vi "BuildingGreyLevelDataBase.vi"(8 "error in (no error)":errorcluster, 9 "ConfDB":T1={"NumberOfImages"=0, "NoImages2SaveAroundFreeze"=0, "Path"=path "", "NameOfPartialFile"="", "StartIndex"=0, "NumberOfStdTol"=0, "Detla t (sec)"=0, "Number of images for baseline"=10, "Temperature File Name"="", "Score"=15.0, "Index number of Files"=[]}, 10 "Droplet Bounding Box":cluster{"x":sgl, "y":sgl}[][](array[cluster]), 11 "Image Ref In":T2) -> (0 "error out":errorcluster, 1 "GreyLevel Drops and time":dbl[][](array[numeric]), 2 "Rel Time (s)":u32[](array[numeric]), 3 "Refnum out":T2(plugin-control), 4 "Greylevel deriv per drop per time":dbl[][](array[numeric]))   [LabVIEW 2013]
doc: "Go over all images and retrieve Grey level of each drop and the difference between the i+1 and i image"
uses:
  <vilib>/vision/Image Controls.llb/IMAQ Image.ctl
  DB/ConfDB.ctl
panel:
  out "Numeric":i32
  out "Index":i32
  out "Time(s)":i32
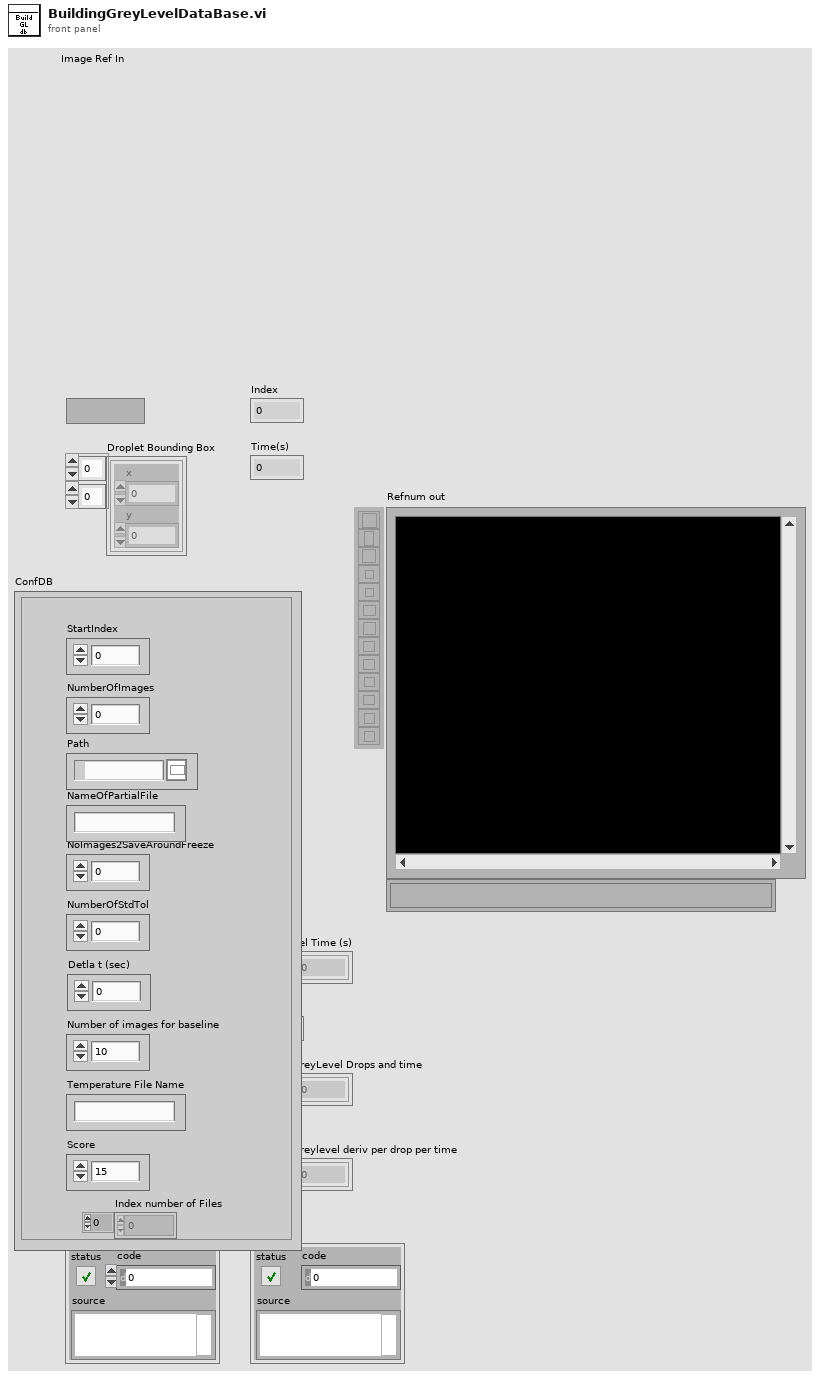
[diagram p1: front panel]
types:
  T1 = typedef "ConfDB.ctl" = cluster{"NumberOfImages":i32, "NoImages2SaveAroundFreeze":i32, "Path":path, "NameOfPartialFile":string, "StartIndex":i32, "NumberOfStdTol":i32, "Detla t (sec)":i32, "Number of images for baseline":i32, "Temperature File Name":string, "Score":dbl, "Index number of Files":i32[]}
  T2 = typedef "IMAQ Image.ctl" = refnum<image>
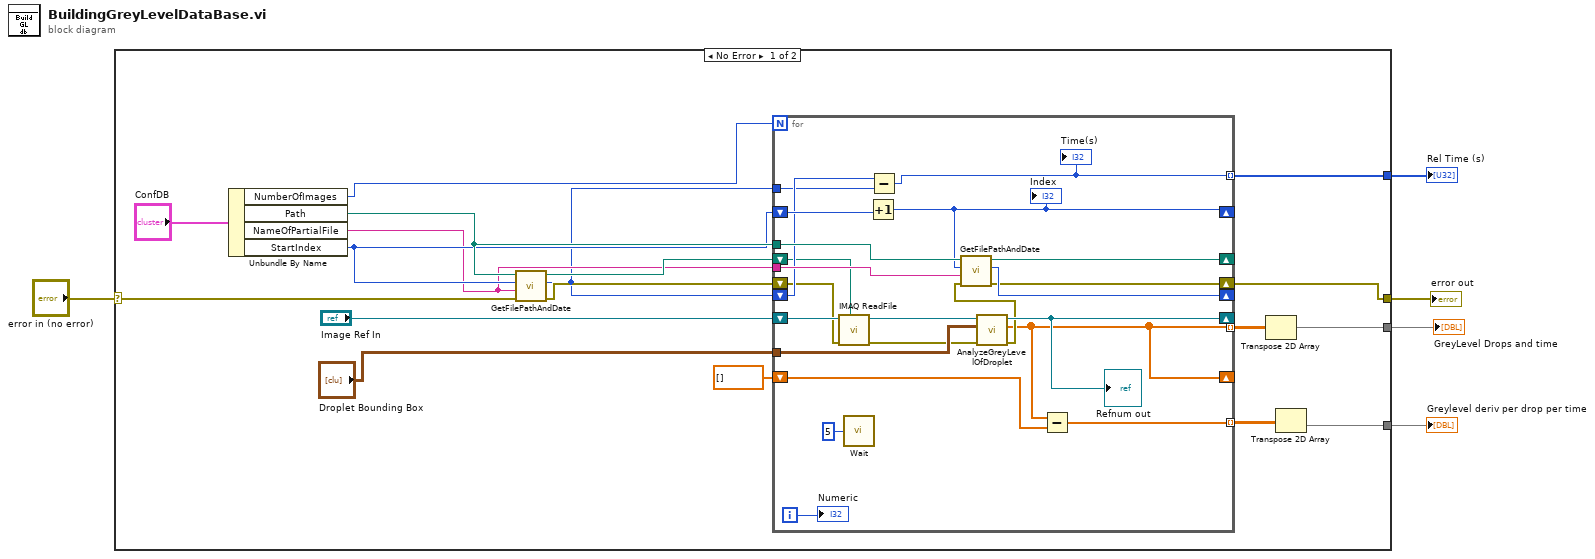
[diagram p0: block diagram]
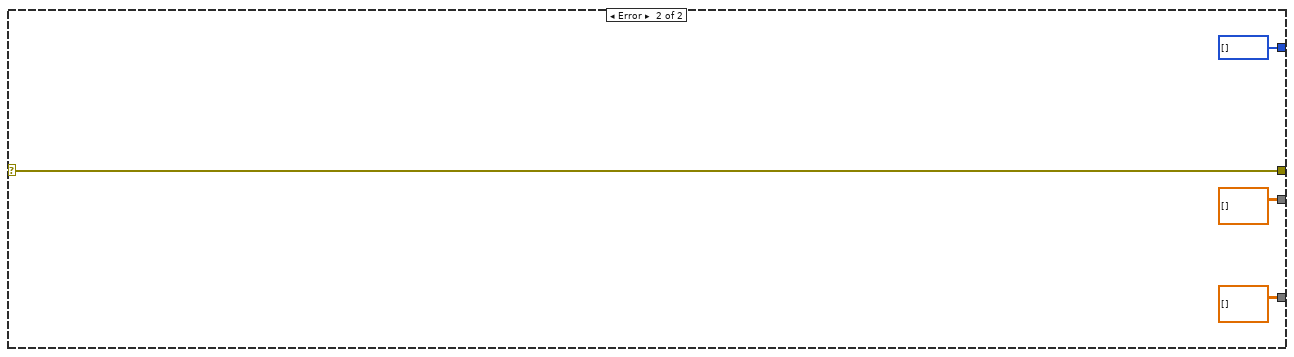
[diagram p2: hidden frame]
diagram:
  n1 = case shown="No Error" "error in (no error)" {
    selector: "error in (no error)" -> [w8 w48]
    tunnel: [w23 dbl[][] []] -> w5
    tunnel: [w21 u32[] []] -> w4
    tunnel: [w19 dbl[][] []] -> w3
    tunnel: [w7 w48] -> w1
    frame No Error {
      n2 = Unbundle By Name("ConfDB") -> ("NumberOfImages"=w18:i32, "Path"=w15:path, "NameOfPartialFile"=w10:string, "StartIndex"=w11:i32)
      n3 = call "GetFilePathAndDate.vi"("error in (no error)"=w8, "String"=w10, "Index"=w11, "Path"=w15) -> ("error out"=w17:errorcluster, "creation date"=w9:u32, "file out"=w14:path)  [unwired: 5 in]
      n4 = for {
        N: w18 -> [_]
        shift-right: [w42] -> _
        shift-left: w11 -> [w46]
        tunnel: [w45] -> w21 mode=indexing
        tunnel: w15 -> [w44]
        tunnel: w10 -> [w43]
        shift-right: [w41] -> _
        shift-left: w14 -> [w35]
        shift-right: [w40] -> _
        shift-left: w9 -> [w39]
        tunnel: w9 -> [w32]
        tunnel: "Droplet Bounding Box" -> [w37]
        shift-right: [w31] -> _
        shift-left: "Image Ref In" -> [w36]
        tunnel: [w26] -> w20 mode=indexing
        shift-right: [w26] -> _
        shift-left: dbl[] [] ("GreyLevelArray") -> [w25]
        shift-right: [w27] -> w7
        shift-left: w17 -> [w30]
        tunnel: [w24] -> w22 mode=indexing
        i -> [w33]
        n5 = call "IMAQ ReadFile"("File Path"=w35, "error in (no error)"=w30, "Image"=w36) -> ("error out"=w29:errorcluster, "Image Out"=w34:T2)  [unwired: 2 in, 5 out]
        n6 = call "Wait"("Count(mSec)"=u32 5) -> ()  [unwired: 1 out]
        n7 = Increment(x=w46) -> (x+1=w42:i32)
        "Index" <- w42
        n8 = Subtract(x=w39, y=w32) -> (x-y=w45:u32)
        "Time(s)" <- w45
        n9 = call "AnalyzeGreyLevelOfDroplet.vi"("error in (no error)"=w29, "Bounding Box"=w37, "Image In"=w34) -> ("error out"=w28:errorcluster, "GreyLevelArray"=w26:dbl[], "Image Out"=w31:T2)  [unwired: 6 in]
        "Refnum out" <- w31
        n10 = call "GetFilePathAndDate.vi"("error in (no error)"=w28, "String"=w43, "Index"=w42, "Path"=w44) -> ("error out"=w27:errorcluster, "creation date"=w40:u32, "file out"=w41:path)  [unwired: 5 in]
        n11 = Subtract(x=w26, y=w25) -> (x-y=w24:dbl[])
        "Numeric" <- w33
      }
      n12 = Transpose 2D Array(2D array=w20) -> (transposed array=w19:dbl[][])
      n13 = Transpose 2D Array(2D array=w22) -> (transposed array=w23:dbl[][])
    }
    frame Error {
    }
  }
  "Greylevel deriv per drop per time" <- w5
  "Rel Time (s)" <- w4
  "GreyLevel Drops and time" <- w3
  "error out" <- w1
